vi "getColumnNames.vi"(8 "error in (no error)":errorcluster, 10 "tableName":string, 11 "schema":string) -> (0 "error out":errorcluster, 2 "columnNamesForQuery":string[](array[string]), 3 "columnNames":string[](array[string]))   [LabVIEW 2023, in "Data Analysis.lvlib"]
uses:
  Data Analysis.lvlib
  HardwareAbstractionLayer_LVOOP/Database/Database.lvclass
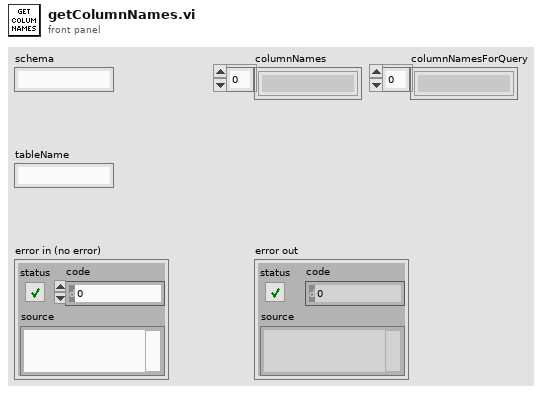
[diagram p1: front panel]
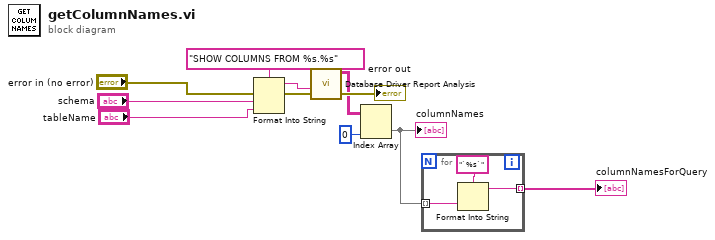
[diagram p0: block diagram]
diagram:
  n1 = Format Into String(format string="SHOW COLUMNS FROM %s.%s" ("SQL query"), error in="error in (no error)", "schema", "tableName") -> (resulting string=w7:string, error out=w6:errorcluster)  [unwired: 1 in]
  n2 = call "Database Driver Report Analysis.vi"("error in"=w6, "SQL query"=w7) -> ("error out"=→"error out":errorcluster, "data"=w8:string[][])  [unwired: 6 in, 2 out]
  n3 = Index Array(array=w8, index (col)=0 ("disabled index (col)")) -> (element=w2:string[])  [unwired: 1 in]
  "columnNames" <- w2
  n4 = for {
    tunnel: w2 -> [w14] mode=indexing
    tunnel: [w12] -> w1 mode=indexing
    n5 = Format Into String(format string="`%s`", w14) -> (resulting string=w12:string)  [unwired: 2 in, 1 out]
  }
  "columnNamesForQuery" <- w1
